vi "Finish.vi"(8 "error in (no error)":errorcluster, 11 "Process In":refnum<class "Debug View.lvclass">) -> (0 "error out":errorcluster, 3 "Process Out":refnum<class "Debug View.lvclass">)   [LabVIEW 2020]
uses:
  Debug View.lvclass
  Public/Lifecycle/Lifecycle State.ctl
  Debug View.lvclass/Debug View.ctl
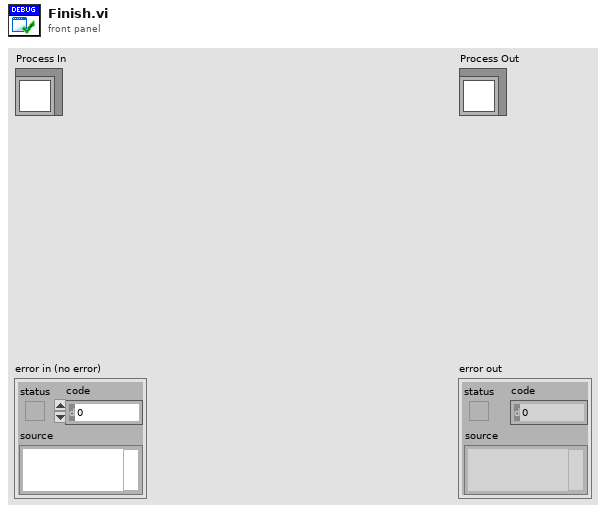
[diagram p1: front panel]
types:
  T1 = typedef "Lifecycle State.ctl" = enum16{"Uninitialized", "Initialized", "Started", "Running", "Stopped", "Finished"}
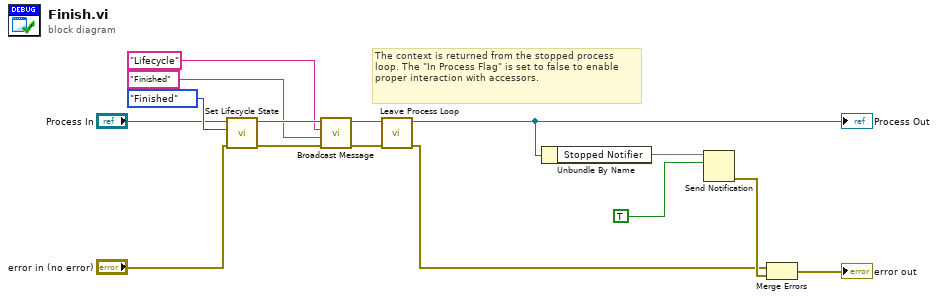
[diagram p0: block diagram]
diagram:
  # "The context is returned from the stopped process loop. The \"In Process Flag\" is set to false to enable proper interaction with accessors."
  n1 = call "Set Lifecycle State.vi"("error in (no error)"="error in (no error)", "Lifecycle State"=Lifecycle_State."Finished", "Process In"="Process In") -> ("error out"=w12:errorcluster, "Process Out"=w13:refnum<class "Debug View.lvclass">)  [unwired: 7 in]
  n2 = call-dynamic "Broadcast Message.vi"("error in (no error)"=w12, "Message Data"="Finished" ("Message"), "Message"="Lifecycle", "Process In"=w13) -> ("error out"=w3:errorcluster, "Process Out"=w5:refnum<class "Debug View.lvclass">)  [unwired: 6 in]
  n3 = call "Leave Process Loop.vi"("error in (no error)"=w3, "Process In"=w5) -> ("error out"=w2:errorcluster, "Process Out"=w4:refnum<class "Debug View.lvclass">)  [unwired: 8 in]
  "Process Out" <- w4
  n4 = Unbundle By Name(w4) -> ("Stopped Notifier"=w15)
  n5 = Send Notification(notification=TRUE, notifier=w15) -> (error out=w8:errorcluster)  [unwired: 1 in, 1 out]
  n6 = Merge Errors(w2, w8) -> (→"error out":errorcluster)
